vi "NIMAXOperation.vi"(8 "error in (no error)":errorcluster, 9 "On/Off":bool=TRUE, 10 "Operation":T1(ring)) -> (0 "error out":errorcluster)   [LabVIEW 2017]
panel:
  in  "Stop Button":bool
  out "Current":dbl
  in  "DAQmx Device Name":tag
  # "V 0.0.a"
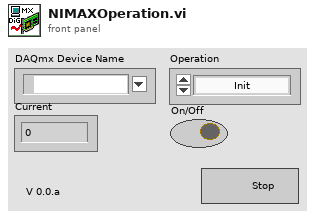
[diagram p1: front panel]
types:
  T1 = enum16{"Init", "0 ohm", "6 ohm", "13.2 ohm", "15 ohm", "25.9 ohm", "33 ohm", "Down", "Up", "Venable", "Firmware", "PowerSuply"}
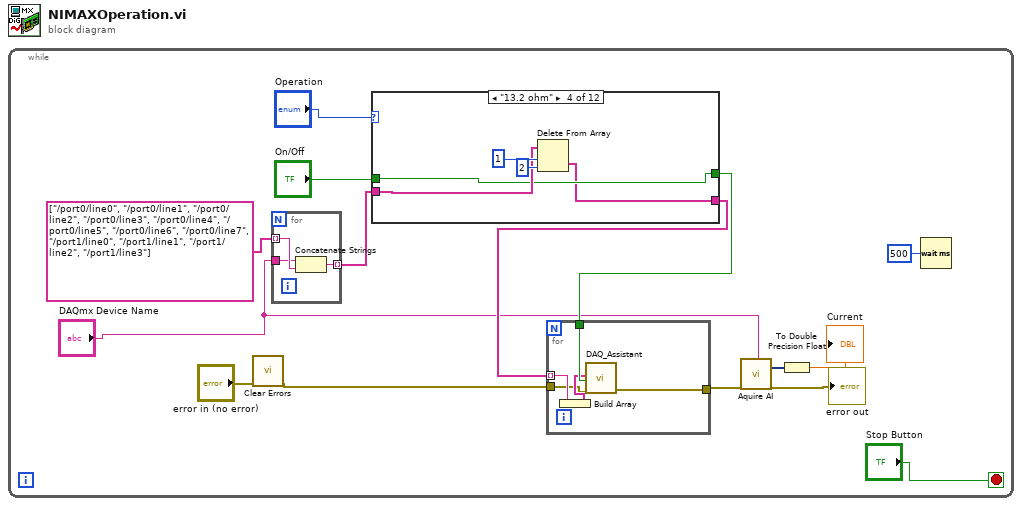
[diagram p0: block diagram]
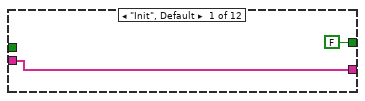
[diagram p2: hidden frame]
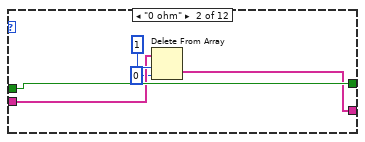
[diagram p3: hidden frame]
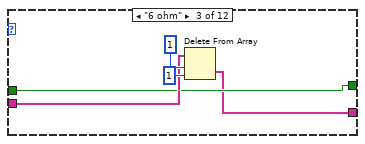
[diagram p4: hidden frame]
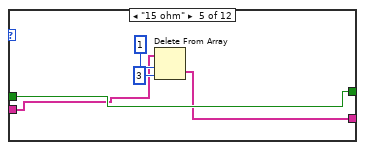
[diagram p5: hidden frame]
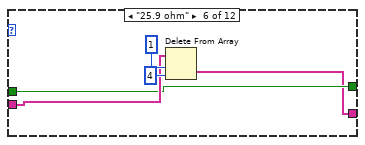
[diagram p6: hidden frame]
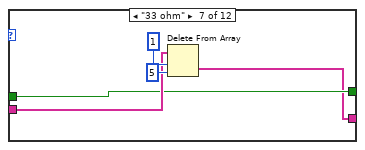
[diagram p7: hidden frame]
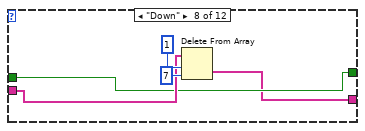
[diagram p8: hidden frame]
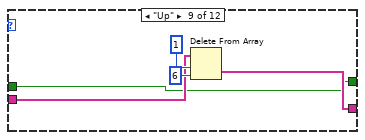
[diagram p9: hidden frame]
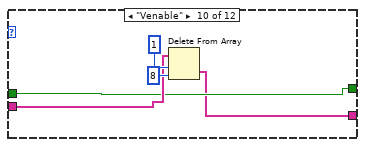
[diagram p10: hidden frame]
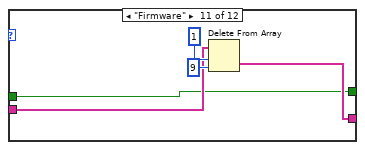
[diagram p11: hidden frame]
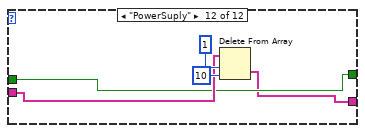
[diagram p12: hidden frame]
diagram:
  n1 = while {
    stop <- "Stop Button" stop-if-true
    n2 = call <vilib>:"Clear Errors.vi"("error in (no error)"="error in (no error)") -> ("error out"=w8:errorcluster)  [unwired: 5 in, 1 out]
    n3 = for {
      tunnel: string[] ["/port0/line0", "/port0/line1", "/port0/line2", "/port0/line3", "/port0/line4", "/port0/line5", "/port0/line6", "/port0/line7", "/port1/line0", "/port1/line1", "/port1/line2", "/port1/line3"] -> [w23] mode=indexing
      tunnel: "DAQmx Device Name" -> [w22]
      tunnel: [w21] -> w9 mode=indexing
      n4 = Concatenate Strings(w22, w23) -> (w21:string)
    }
    n5 = case shown="\"13.2 ohm\"" "Operation" {
      tunnel: "On/Off" -> [_ w30 w32 w37 w43 w47 w52 w57 w61 w67 w71 w77]
      tunnel: [FALSE ("On/Off") w30 w32 w37 w43 w47 w52 w57 w61 w67 w71 w77] -> w12
      tunnel: [w24 w26 w31 w36 w41 w46 w51 w56 w62 w66 w72 w76] -> w11
      tunnel: w9 -> [w24 w28 w33 w38 w42 w48 w53 w58 w63 w68 w73 w78]
      frame "Init", Default {
      }
      frame "0 ohm" {
        n6 = Delete From Array(array=w28, length=1, index=0) -> (deleted portion=w26:string[])  [unwired: 1 out]
      }
      frame "6 ohm" {
        n7 = Delete From Array(array=w33, length=1, index=1) -> (deleted portion=w31:string[])  [unwired: 1 out]
      }
      frame "13.2 ohm" {
        n8 = Delete From Array(array=w38, length=1, index=2) -> (deleted portion=w36:string[])  [unwired: 1 out]
      }
      frame "15 ohm" {
        n9 = Delete From Array(array=w42, length=1, index=3) -> (deleted portion=w41:string[])  [unwired: 1 out]
      }
      frame "25.9 ohm" {
        n10 = Delete From Array(array=w48, length=1, index=4) -> (deleted portion=w46:string[])  [unwired: 1 out]
      }
      frame "33 ohm" {
        n11 = Delete From Array(array=w53, length=1, index=5) -> (deleted portion=w51:string[])  [unwired: 1 out]
      }
      frame "Down" {
        n12 = Delete From Array(array=w58, length=1, index=7) -> (deleted portion=w56:string[])  [unwired: 1 out]
      }
      frame "Up" {
        n13 = Delete From Array(array=w63, length=1, index=6) -> (deleted portion=w62:string[])  [unwired: 1 out]
      }
      frame "Venable" {
        n14 = Delete From Array(array=w68, length=1, index=8) -> (deleted portion=w66:string[])  [unwired: 1 out]
      }
      frame "Firmware" {
        n15 = Delete From Array(array=w73, length=1, index=9) -> (deleted portion=w72:string[])  [unwired: 1 out]
      }
      frame "PowerSuply" {
        n16 = Delete From Array(array=w78, length=1, index=10) -> (deleted portion=w76:string[])  [unwired: 1 out]
      }
    }
    n17 = for {
      tunnel: w11 -> [w18] mode=indexing
      tunnel: w12 -> [w20]
      tunnel: [w19] -> w7
      tunnel: w8 -> [w16]
      n18 = Build Array(w18) -> (w17:string[])
      n19 = call "DAQ_Assistant.vi"("Lines"=w17, "data 2"=w20, "error in"=w16) -> ("error out"=w19:errorcluster)  [unwired: 15 in, 1 out]
    }
    n20 = call "Aquire AI"("error in"=w7, "device name"="DAQmx Device Name") -> ("data"=w4:dynamicdata, "error out"=→"error out":errorcluster)  [unwired: 15 in, 1 out]
    n21 = To Double Precision Float(number=w4) -> (double precision float=→"Current":dbl)
    n22 = Wait (ms)(milliseconds to wait=u32 500) -> ()  [unwired: 1 out]
  }
